vi "stop_vlc_1.vi"(8 "error in (no error)":errorcluster, 9 "Timeout (ms)":i32) -> (0 "error out":errorcluster)   [LabVIEW 2018]
panel:
  out "Open Proceesses":string[](array[string])=["C:\\Program Files\\National Instruments\\LabVIEW 8.2\\LabVIEW.exe"]
  out "Loops":i32
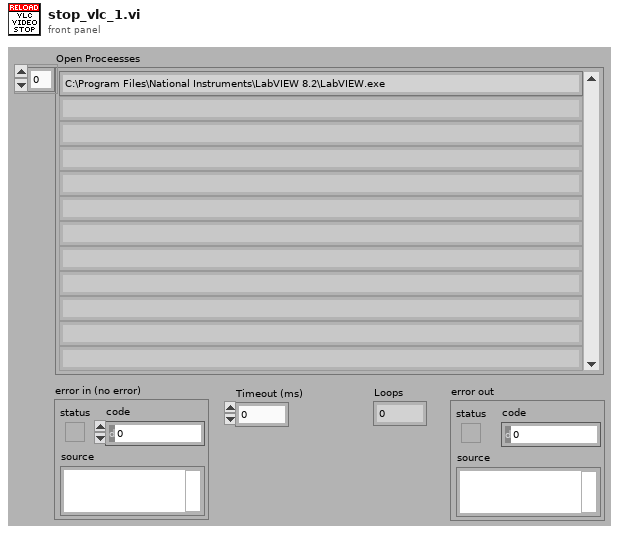
[diagram p1: front panel]
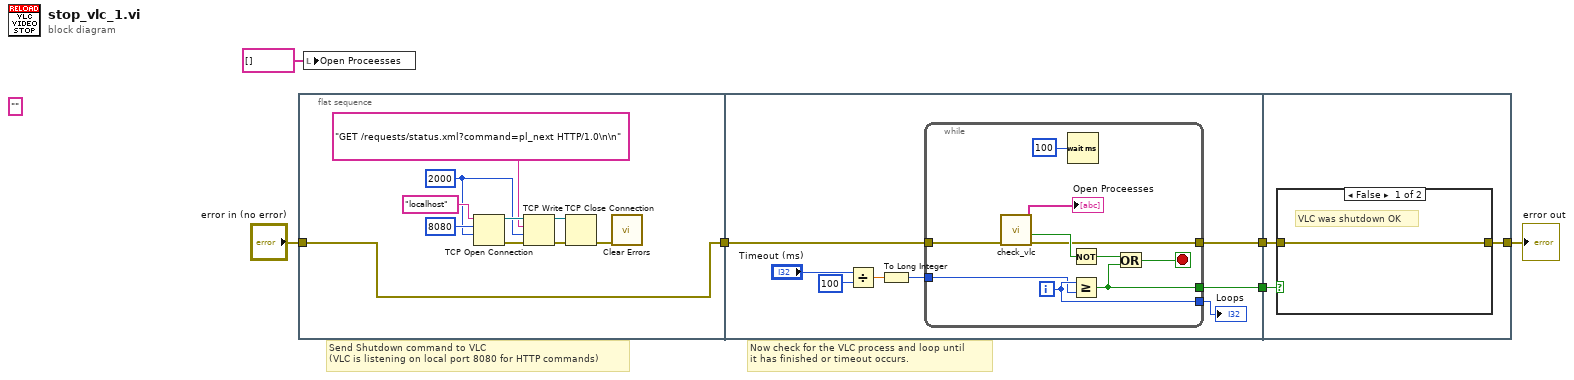
[diagram p0: block diagram]
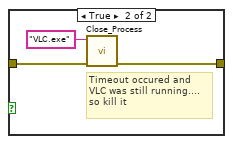
[diagram p2: hidden frame]
diagram:
  (unwired) "" ("ModuleName")
  # "Now check for the VLC process and loop until\nit has finished or timeout occurs."
  # "Send Shutdown command to VLC\n(VLC is listening on local port 8080 for HTTP commands)"
  n1 = flat-sequence {
    tunnel: "error in (no error)" -> [w8]
    tunnel: [w8] -> w4
    tunnel: [w20] -> w6
    tunnel: w4 -> [w18]
    tunnel: [w17] -> w3
    tunnel: w6 -> [w37]
    tunnel: w3 -> [w36]
    tunnel: [w35] -> w2
    frame #0 {
      w10 = u16 2000 ("remote port")
      n2 = TCP Open Connection(address="localhost" ("Address"), remote port or service name=u16 8080 ("remote port"), timeout ms (60000)=w10) -> (connection ID=w13:refnum<k5>, error out=w16:errorcluster)  [unwired: 1 in, 1 out]
      n3 = TCP Write(connection ID=w13, data in="GET /requests/status.xml?command=pl_next HTTP/1.0\n\n", error in (no error)=w16, 9:w10) -> (connection ID out=w11:refnum<k5>, error out=w12:errorcluster)  [unwired: 1 out]
      n4 = TCP Close Connection(connection ID=w11, error in (no error)=w12) -> (error out=w7:errorcluster)  [unwired: 2 out]
      n5 = call <vilib>:"Clear Errors.vi"("error in (no error)"=w7) -> ()  [unwired: 1 in, 6 out]
    }
    frame #1 {
      n6 = Divide(x="Timeout (ms)", y=100) -> (x/y=w22:dbl)
      n7 = To Long Integer(number=w22) -> (32bit integer=w21:i32)
      n8 = while {
        tunnel: w21 -> [w28]
        tunnel: [w31] -> w20
        tunnel: [w29] -> w19
        tunnel: w18 -> [w27]
        tunnel: [w26] -> w17
        i -> [w29]
        stop <- w32 stop-if-true
        n9 = call "check_vlc.vi"("error in (no error)"=w27) -> ("error out"=w26:errorcluster, "Match?"=w33:bool, "Open Proceesses"=→"Open Proceesses":string[])  [unwired: 8 out]
        n10 = Wait (ms)(milliseconds to wait=u32 100) -> ()  [unwired: 1 out]
        n11 = Not(x=w33) -> (.not. x?=w30:bool)
        n12 = Greater Or Equal?(x=w29, y=w28) -> (x >= y?=w31:bool)
        n13 = Or(x=w30, y=w31) -> (x .or. y?=w32:bool)
      }
      "Loops" <- w19
    }
    frame #2 {
      n14 = case shown="False" w37 {
        tunnel: w36 -> [w38 w40]
        tunnel: [w38 w39] -> w35
        frame False {
          # "VLC was shutdown OK"
        }
        frame True {
          # "Timeout occured and\nVLC was still running....\nso kill it"
          n15 = call "Close_Process.vi"("error in (no error)"=w40, "Process to kill"="VLC.exe") -> ("error out"=w39:errorcluster)  [unwired: 9 out]
        }
      }
    }
  }
  n16 = local write "Open Proceesses"(string[] [] ("Open Proceesses")) -> ()
  "error out" <- w2
